vi "TIO RPC Notification U32.vi"(4 "Notification Prefix":string, 7 "error in (no error)":errorcluster, 8 "U32":u32, 9 "Read":bool, 10 "String":string) -> (0 "error out":errorcluster, 1 "U32 Returned (default if error)":u32, 2 "Response":bool)   [LabVIEW 2017]
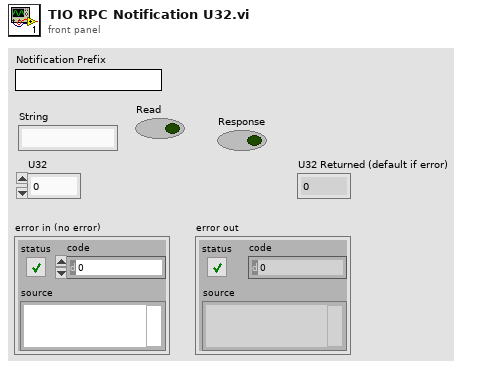
[diagram p1: front panel]
types:
  T1 = enum16{"big-endian, network order", "native, host order", "little-endian"}
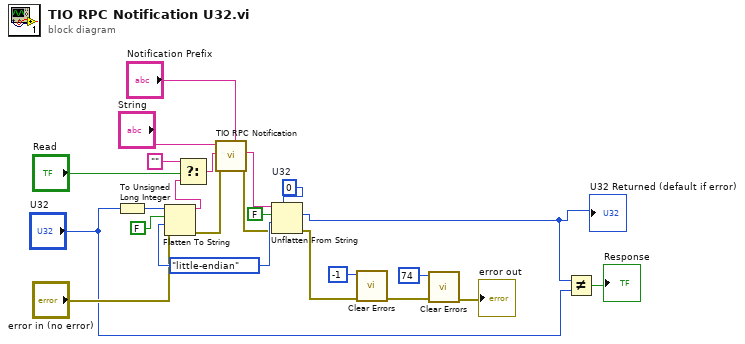
[diagram p0: block diagram]
diagram:
  w23 = u32 0  # U32
  w20 = T1."little-endian" ("byte order (0:big-endian, network order)")
  n1 = To Unsigned Long Integer(number="U32") -> (unsigned 32bit integer=w15:u32)
  n2 = Flatten To String(anything=w15, prepend array or string size? (T)=FALSE, byte order (0:big-endian, network order)=w20, error in (no error)="error in (no error)") -> (data string=w17:string, error out=w11:errorcluster)  [unwired: 1 out]
  n3 = Select(t="", s="Read", f=w17) -> (s? t:f=w16:string)
  n4 = call <instrlib>:"TIO RPC Notification.vi"("Notification Prefix"="Notification Prefix", "error in (no error)"=w11, "Payload"=w16, "Topic"="String") -> ("error out"=w3:errorcluster, "REP"=w21:string)  [unwired: 4 in, 1 out]
  n5 = Unflatten From String(type=w23, binary string=w21, data includes array or string size? (T)=FALSE, byte order (0:big-endian, network order)=w20, error in (no error)=w3) -> (value=w1:u32, error out=w7:errorcluster)  [unwired: 1 out]
  "U32 Returned (default if error)" <- w1
  n6 = call <vilib>:"Clear Errors.vi"("error in (no error)"=w7, "specific error code to clear (0: all)"=-1) -> ("error out"=w9:errorcluster)  [unwired: 4 in, 1 out]
  n7 = call <vilib>:"Clear Errors.vi"("error in (no error)"=w9, "specific error code to clear (0: all)"=74) -> ("error out"=→"error out":errorcluster)  [unwired: 4 in, 1 out]
  n8 = Not Equal?(x=w1, y="U32") -> (x != y?=→"Response":bool)
